vi "メイン_測定値配列_CSV転記サブ.vi"(7 "メイン設定_設定入力":T1 {"測定モード" items=["単発測定モード", "連続測定モード", "多点測定モード"]}, 8 "ループ反復数値入力":i32, 9 "実測設定項目":T1 {"測定モード" items=["単発測定モード", "連続測定モード", "多点測定モード"]}, 10 "使用ON/OFF":bool, 11 "前回値転記用配列":refnum<vi>) -> (2 "ループ反復数値出力":i32, 3 "メイン設定_設定出力":T1 {"測定モード" items=["単発測定モード", "連続測定モード", "多点測定モード"]})   [LabVIEW 2021]
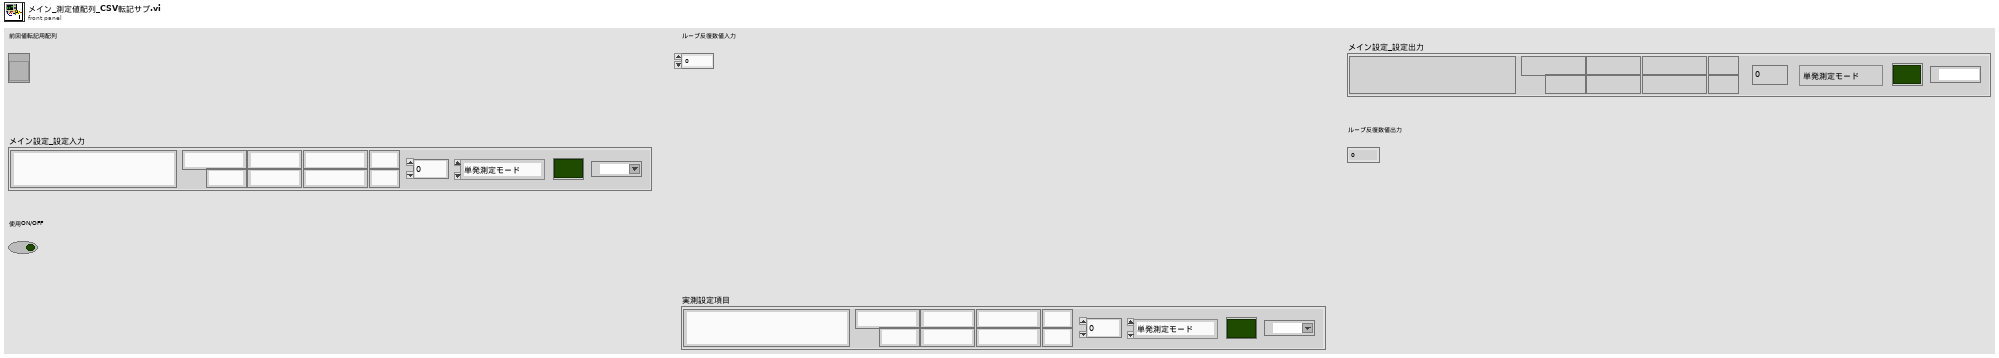
[diagram p1: front panel]
types:
  T1 = typedef "設定全項目制御器.ctl" = cluster{"規格":string, "規格上限":string, "規格下限":string, "ポートNo.":dbl, "測定モード":u16, "規格単位":string, "品質チェック項目":string, "測定周期":dbl, "実測値MAX":string, "実測値MIN":string, "実測値(MAX)":string, "実測値(MIN)":string, "測定画面表示ボタン":bool, "ゲージポートNo":refnum<visa-resource-name>}
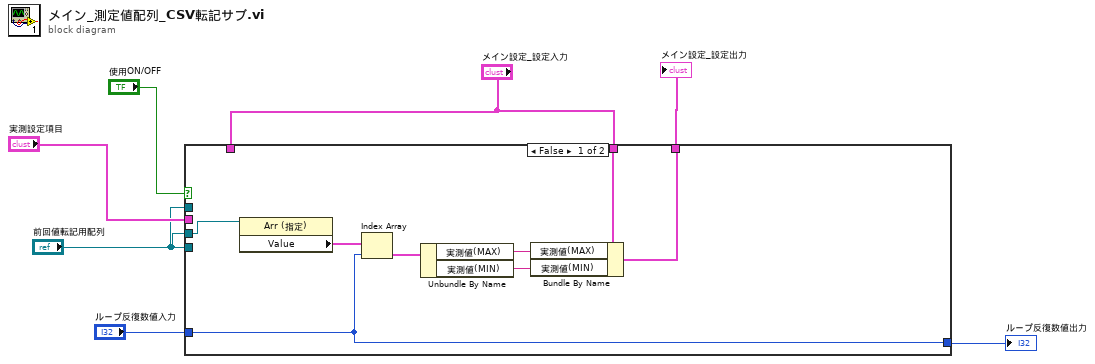
[diagram p0: block diagram]
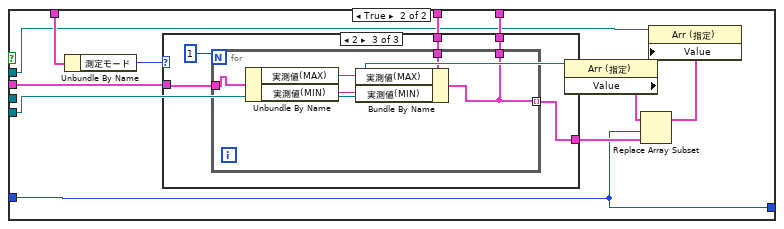
[diagram p2: hidden frame]
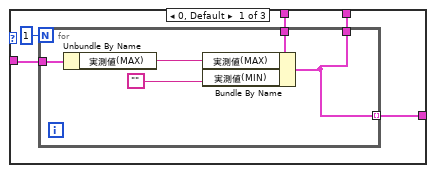
[diagram p3: hidden frame]
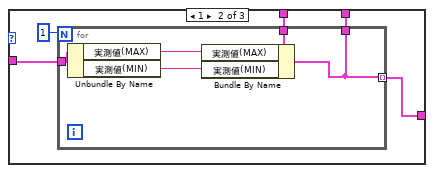
[diagram p4: hidden frame]
diagram:
  n1 = case shown="FALSE" "使用ON/OFF" {
    tunnel: "実測設定項目" -> [_ w25]
    tunnel: "ループ反復数値入力" -> [w9 w18]
    tunnel: "メイン設定_設定入力" -> [_ w24]
    tunnel: [w14 w23] -> w5
    tunnel: "メイン設定_設定入力" -> [w15 w22]
    tunnel: [w9 w18] -> w7
    tunnel: "前回値転記用配列" -> [w8 _]
    tunnel: "前回値転記用配列" -> [_ w17]
    tunnel: "前回値転記用配列" -> [_ w16]
    frame False {
      n2 = property on="プロパティノード" class="Arr (指定)"(reference=w8) -> ("Value"=w13:T1[])  [unwired: 1 in, 2 out]
      n3 = Index Array(array=w13, index=w9) -> (element=w12:T1)
      n4 = Unbundle By Name(w12) -> ("実測値(MAX)"=w11:string, "実測値(MIN)"=w10:string)
      n5 = Bundle By Name(cluster=w15, "実測値(MAX)"=w11, "実測値(MIN)"=w10) -> (w14:T1)
    }
    frame True {
      n6 = Unbundle By Name(w24) -> ("測定モード"=w26:u16)
      n7 = case shown="2" w26 {
        tunnel: w25 -> [w31 w39 w49]
        tunnel: [w29 w40 w50] -> w20
        tunnel: [w27 w37 w48] -> w23
        tunnel: w22 -> [w28 w38 w47]
        frame 0, Default {
          n8 = for {
            N: 1 -> [_]
            tunnel: w31 -> [w36]
            tunnel: [w32] -> w29 mode=indexing
            tunnel: w28 -> [w33]
            tunnel: [w32] -> w27
            n9 = Unbundle By Name(w36) -> ("実測値(MAX)"=w34:string)
            n10 = Bundle By Name(cluster=w33, "実測値(MAX)"=w34, "実測値(MIN)"="") -> (w32:T1)
          }
        }
        frame 1 {
          n11 = for {
            N: 1 -> [_]
            tunnel: [w42] -> w40 mode=indexing
            tunnel: w39 -> [w44]
            tunnel: w38 -> [w43]
            tunnel: [w42] -> w37
            n12 = Unbundle By Name(w44) -> ("実測値(MAX)"=w45:string, "実測値(MIN)"=w46:string)
            n13 = Bundle By Name(cluster=w43, "実測値(MAX)"=w45, "実測値(MIN)"=w46) -> (w42:T1)
          }
        }
        frame 2 {
          n14 = for {
            N: 1 -> [_]
            tunnel: [w53] -> w50 mode=indexing
            tunnel: w49 -> [w54]
            tunnel: [w53] -> w48
            tunnel: w47 -> [w52]
            n15 = Unbundle By Name(w54) -> ("実測値(MAX)"=w55:string, "実測値(MIN)"=w56:string)
            n16 = Bundle By Name(cluster=w52, "実測値(MAX)"=w55, "実測値(MIN)"=w56) -> (w53:T1)
          }
        }
      }
      n17 = property on="プロパティノード" class="Arr (指定)"(reference=w17) -> ("Value"=w21:T1[])  [unwired: 1 in, 2 out]
      n18 = Replace Array Subset(array=w21, new element=w20, index=w18) -> (w19:T1[])
      n19 = property class="Arr (指定)"(reference=w16, "Value"=w19) -> ()  [unwired: 1 in, 2 out]
    }
  }
  "ループ反復数値出力" <- w7
  "メイン設定_設定出力" <- w5
